vi "启动参数写入.vi"(4 "error in (no error)":errorcluster caption="错误输入（无错误）", 5 "Value":T3 caption="值", 6 "Container State":T4 caption="容器状态", 7 "Display State In":T1 caption="显示状态输入") -> (0 "error out":errorcluster caption="错误输出", 3 "Display State Out":T1 caption="显示状态输出")   [LabVIEW 2016, in "调试控件V3.xctl"]
uses:
  <vilib>/_xctls/Container State.ctl
  <vilib>/_xctls/XControlSupport.lvlib
panel:
  # "将以下值显示控件替换为所需类型的显示控件。\n不要从连线板中删除该显示控件或其它显示控件。\n不要更改连线板模式。\n值显示控件应始终位于连线板输出端自顶部起第三个接线端。"
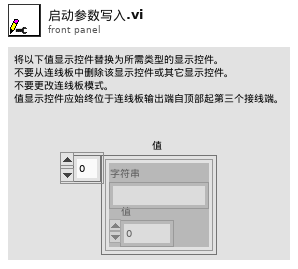
[diagram p1: front panel]
types:
  T1 = typedef "调试控件V3.xctl/状态 2.ctl" = cluster{"仪器类型":T2, "字符串与值[]":T3}
  T2 = typedef "调试控件V3.xctl/仪器类型.ctl" = enum16{"A版", "B版"}
  T3 = typedef "调试控件V3.xctl/启动参数.ctl" = cluster{"String":string, "Value":u16}[]
  T4 = typedef "XControlSupport.lvlib/Container State.ctl" = cluster{"Indicator?":bool, "Run Mode?":bool, " Refnum":refnum<vi>}
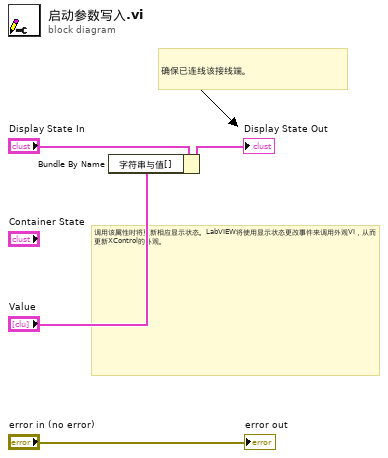
[diagram p0: block diagram]
diagram:
  # "确保已连线该接线端。"
  # "调用该属性时将更新相应显示状态。LabVIEW将使用显示状态更改事件来调用外观VI，从而更新XControl的外观。"
  n1 = Bundle By Name(cluster="Display State In", "字符串与值[]"="Value") -> (→"Display State Out":T1)
  "error out" <- "error in (no error)"
